vi "Status Get Pressure and Flow Rate.vi"(5 "Retry Attempts (0)":i32 min=0, 8 "error in":errorcluster, 11 "VISA resource name":refnum<visa-resource-name>) -> (0 "error out":errorcluster, 1 "Flow Rate":dbl, 2 "Pressure":i32, 3 "VISA resource name out":refnum<visa-resource-name>)   [LabVIEW 2020, in "ChromTech Series III Pump.lvlib"]
doc: "Queries the pump for current conditions of pressure and flow rate."
uses:
  <instrlib>/RxnRover/ChromtechSeriesIIIDriver/ChromTech Series III Pump.lvlib
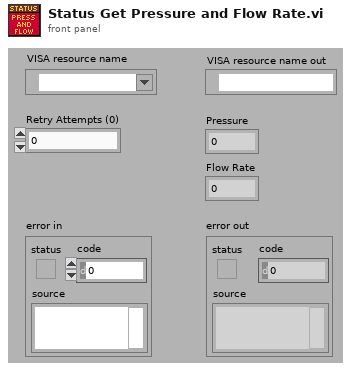
[diagram p1: front panel]
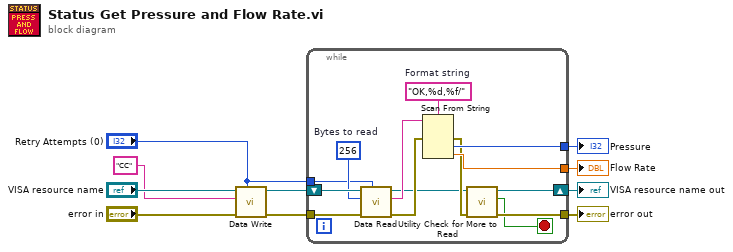
[diagram p0: block diagram]
diagram:
  n1 = call <instrlib>:"Data Write.vi"("Retry Attempts (0)"="Retry Attempts (0)", "error in (no error)"="error in", "Command"="CC", "VISA Refnum in"="VISA resource name") -> ("error out"=w7:errorcluster, "VISA Refnum out"=w6:refnum<visa-resource-name>)  [unwired: 6 in]
  n2 = while {
    tunnel: [w20] -> w5
    tunnel: [w19] -> w4
    tunnel: "Retry Attempts (0)" -> [w15]
    shift-right: [w12] -> w2
    shift-left: w6 -> [w23]
    tunnel: w7 -> [w24]
    tunnel: [w14] -> w3
    stop <- w11 stop-if-true
    w21 = "OK,%d,%f/"  # Format string
    w22 = u32 256  # Bytes to read
    n3 = call <instrlib>:"Data Read.vi"("Retry Attempts (0)"=w15, "error in (no error)"=w24, "Bytes to read"=w22, "VISA Refnum in"=w23) -> ("error out"=w18:errorcluster, "read buffer"=w16:string, "VISA Refnum out"=w13:refnum<visa-resource-name>)  [unwired: 5 in]
    n4 = Scan From String(format string=w21, input string=w16, error in=w18) -> (error out=w17:errorcluster, output 1=w20:i32, output 2=w19:dbl)  [unwired: 3 in, 2 out]
    n5 = call <instrlib>:"Utility Check for More to Read.vi"("error in (no error)"=w17, "VISA Refnum in"=w13) -> ("error out (unchanged)"=w14:errorcluster, "More to read?"=w11:bool, "VISA Refnum out"=w12:refnum<visa-resource-name>)  [unwired: 7 in]
  }
  "VISA resource name out" <- w2
  "error out" <- w3
  "Pressure" <- w5
  "Flow Rate" <- w4
